vi "Handle Last Ack Core.vi"(4 "error in (no error)":errorcluster, 6 "Last Ack":refnum<class "Last Ack.lvclass">, 7 "State Machine in":refnum<class "State Machine.lvclass">) -> (0 "error out":errorcluster, 3 "State Machine out":refnum<class "State Machine.lvclass">)   [LabVIEW 2024, in "State Pattern Actor.lvlib" / "State Machine.lvlib" / "State Machine.lvclass"]
doc: "<p>(<strong>Filename</strong>: <span class=\"dnl\">Actor Framework.lvlib:Actor.lvclass:Handle Last Ack Core.vi</span>)</p>\n<p>Defines how the caller actor responds to the Last Ack message from a nested actor. The Last Ack message is the final message a nested actor sends to its caller before it shuts down. The message contains information about the final state of the nested actor.</p>\n<p>By default, this method does nothing except return any error the nested actor sent. A descendant class may override this method to define behavior.</p>"
uses:
  State Machine.lvclass
  State Machine.lvclass/State Machine.ctl
  <vilib>/ActorFramework/Actor/Actor.lvclass
  <vilib>/ActorFramework/LastAck/Last Ack.lvclass
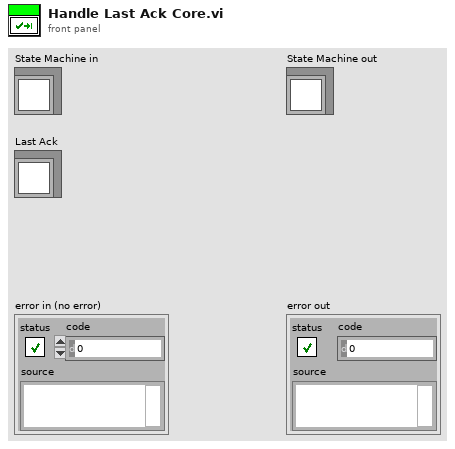
[diagram p1: front panel]
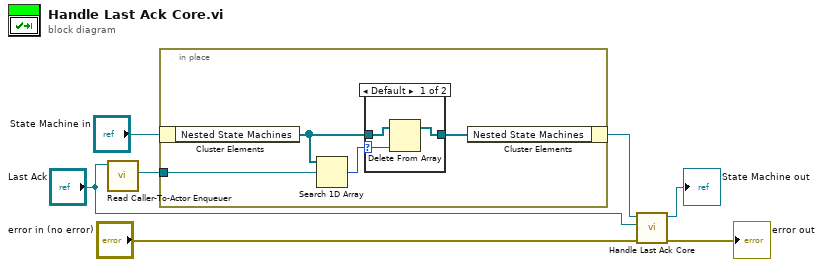
[diagram p0: block diagram]
diagram:
  n1 = call <vilib>:"Read Caller-To-Actor Enqueuer.vi"("Last Ack"="Last Ack") -> ("Caller-to-Actor Enqueuer"=w3:refnum<class "Message Enqueuer.lvclass">)  [unwired: 10 in]
  n2 = in-place {
    in-place-border: w3 -> [w11]
    n3 = in-place-cluster #1("State Machine in") -> ("Nested State Machines"=w8:refnum<class "Message Enqueuer.lvclass">[])
    n4 = Search 1D Array(1D array=w8, element=w11) -> (index of element=w10:i32)  [unwired: 1 in]
    n5 = case shown="Default" w10 {
      selector: w10 -> [w12 _]
      tunnel: [w13 w15] -> w9
      tunnel: w8 -> [w14 w15]
      frame Default {
        n6 = Delete From Array(array=w14, index=w12) -> (array with subset deleted=w13:refnum<class "Message Enqueuer.lvclass">[])  [unwired: 1 in, 1 out]
      }
      frame -1 {
      }
    }
    n7 = in-place-cluster #1("Nested State Machines"=w9) -> (w1:refnum<class "State Machine.lvclass">)
  }
  n8 = call-parent "Handle Last Ack Core.vi"("error in (no error)"="error in (no error)", "Last Ack"="Last Ack", "Actor in"=w1) -> ("error out"=→"error out":errorcluster, "Actor out"=→"State Machine out":refnum<class "State Machine.lvclass">)  [unwired: 3 in]
